vi "Sort Appropriate Subsequences Based on Length and Return Longest.vi"(11 "Appropriate Subsequences":T1[](array[typedef])) -> (3 "Logest Length Subsequence Match":T1)   [LabVIEW 2013, in "GA.lvclass"]
uses:
  GA.lvclass
  Controls/Appropraite Subsequences for SXX.ctl
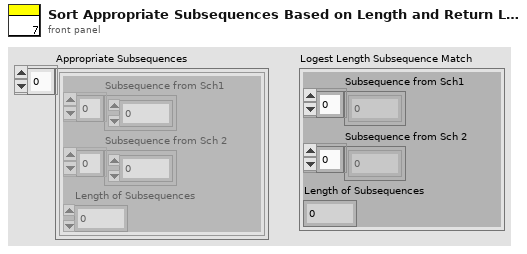
[diagram p1: front panel]
types:
  T1 = typedef "Appropraite Subsequences for SXX.ctl" = cluster{"Subsequence from Sch1":i32[], "Subsequence from Sch 2":i32[], "Length of Subsequences":i32}
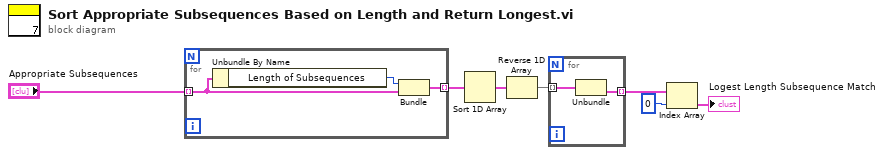
[diagram p0: block diagram]
diagram:
  n1 = for {
    tunnel: "Appropriate Subsequences" -> [w9] mode=indexing
    tunnel: [w8] -> w5 mode=indexing
    n2 = Unbundle By Name(w9) -> ("Length of Subsequences"=w10:i32)
    n3 = Bundle("Length of Subsequences"=w10, w9) -> (w8:cluster{"Length of Subsequences":i32, T1})  [unwired: 1 in]
  }
  n4 = Sort 1D Array(array=w5) -> (sorted array=w4:cluster{"Length of Subsequences":i32, T1}[])
  n5 = Reverse 1D Array(array=w4) -> (reversed array=w3:cluster{"Length of Subsequences":i32, T1}[])
  n6 = for {
    tunnel: w3 -> [w12] mode=indexing
    tunnel: [w11] -> w2 mode=indexing
    n7 = Unbundle(w12) -> (w11:T1)  [unwired: 1 out]
  }
  n8 = Index Array(array=w2, index=0) -> (element=→"Logest Length Subsequence Match":T1)
